vi "Analyze.vi"(8 "error in (no error)":errorcluster, 9 "Work Image":T1, 10 "Destination":refnum<class "Message Enqueuer.lvclass">, 11 "Analyze Data":T2) -> (0 "error out":errorcluster)   [LabVIEW 2014, in "Analyze Actor.lvlib" / "Analyze Actor.lvclass"]
uses:
  Analyze Actor.lvclass
  HIJ Vision Display/HIJ Vision Display/Analyze.ctl
  Abstract Messages/Publish Analyze Results Msg/Publish Analyze Results Msg.lvclass
  <vilib>/vision/Image Controls.llb/IMAQ Image.ctl
  Analyze Classes/Analyze BaseClass/Analyze BaseClass/Analyze BaseClass.lvclass
  Results and Overlays/Results Base/Analyze Results Base.lvclass
  <vilib>/ActorFramework/Message Enqueuer/Message Enqueuer.lvclass
  Abstract Messages/Publish Analyze Results Msg/Publish Analyze Results Msg.lvclass/Publish Analyze Results Msg.ctl
  <vilib>/ActorFramework/Message Enqueuer/Message Enqueuer.lvclass/Message Enqueuer.ctl
  <vilib>/ActorFramework/Message Enqueuer/Enqueue.vi
  <vilib>/ActorFramework/Message Priority Queue/Priority Enqueue.vi
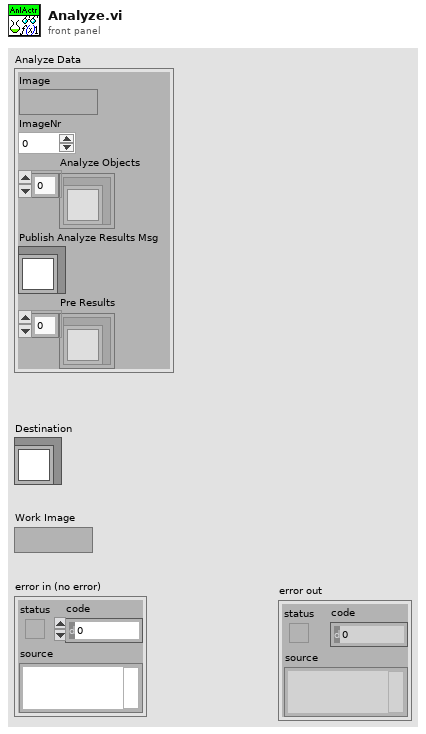
[diagram p1: front panel]
types:
  T1 = typedef "IMAQ Image.ctl" = refnum<image>
  T2 = typedef "Analyze Actor.lvlib/Analyze Actor.lvclass/Analyze.ctl" = cluster{"Image":T1, "ImageNr":i32, "Analyze Objects":refnum<class "Analyze BaseClass.lvclass">[], "Publish Analyze Results Msg":refnum<class "Publish Analyze Results Msg.lvclass">, "Pre Results":refnum<class "Analyze Results Base.lvclass">[]}
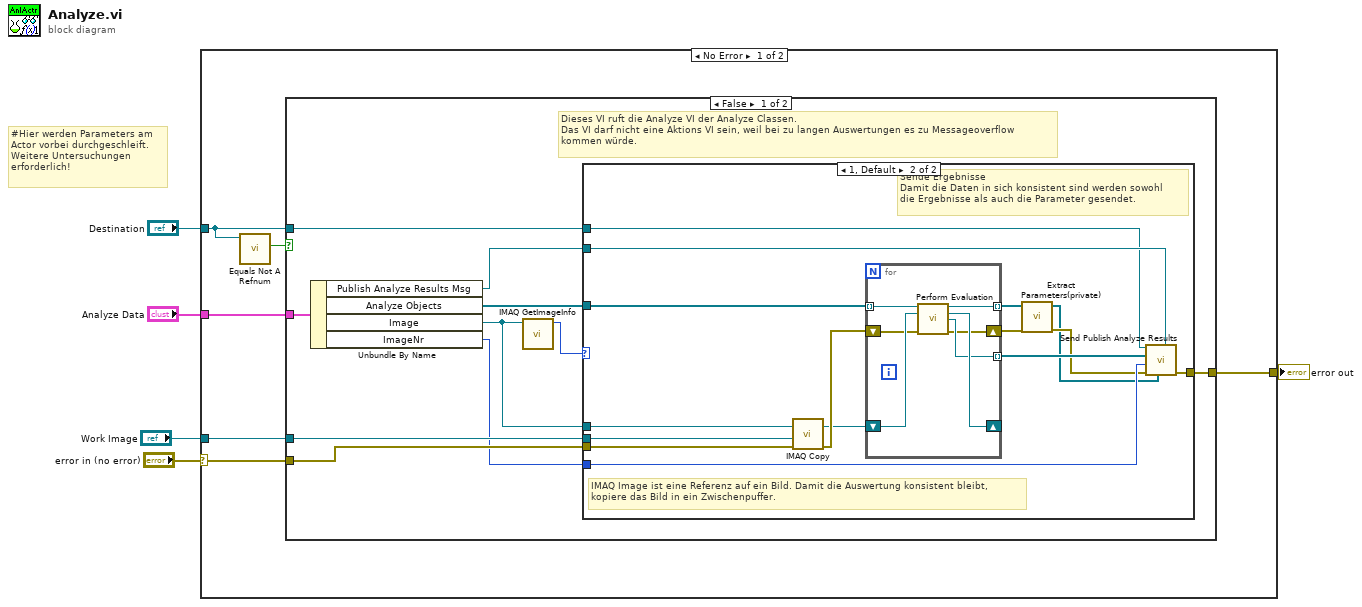
[diagram p0: block diagram]
diagram:
  # "#Hier werden Parameters am\nActor vorbei durchgeschleift.\nWeitere Untersuchungen \nerforderlich!"
  n1 = case shown="No Error" "error in (no error)" {
    selector: "error in (no error)" -> [w11 w46]
    tunnel: [w9 w46] -> w4
    tunnel: "Analyze Data" -> [w10 _]
    tunnel: "Destination" -> [w8 _]
    tunnel: "Work Image" -> [w6 _]
    frame No Error {
      n2 = call <vilib>:"Equals Not A Refnum.vi"("Message Enqueuer"=w8) -> ("Not a refnum?"=w7:bool)  [unwired: 10 in]
      n3 = case shown="False" w7 {
        tunnel: w11 -> [w15 w45]
        tunnel: w10 -> [w20 _]
        tunnel: [w18 w45] -> w9
        tunnel: w8 -> [w17 _]
        tunnel: w6 -> [w16 _]
        frame False {
          # "Dieses VI ruft die Analyze VI der Analyze Classen.\nDas VI darf nicht eine Aktions VI sein, weil bei zu langen Auswertungen es zu Messageoverflow\nkommen würde."
          n4 = Unbundle By Name(w20) -> ("Publish Analyze Results Msg"=w21:refnum<class "Publish Analyze Results Msg.lvclass">, "Analyze Objects"=w19:refnum<class "Analyze BaseClass.lvclass">[], "Image"=w13:T1, "ImageNr"=w14:i32)
          n5 = call "IMAQ GetImageInfo"("Image"=w13) -> ("X Resolution"=w12:i32)  [unwired: 3 in, 7 out]
          n6 = case shown="1, Default" w12 {
            tunnel: w21 -> [_ w37]
            tunnel: w19 -> [_ w36]
            tunnel: [w22 w35] -> w18
            tunnel: w17 -> [_ w34]
            tunnel: w16 -> [_ w33]
            tunnel: w15 -> [w22 w32]
            tunnel: w14 -> [_ w29]
            tunnel: w13 -> [_ w23]
            frame 0 {
            }
            frame 1, Default {
              # "Sende Ergebnisse\nDamit die Daten in sich konsistent sind werden sowohl\ndie Ergebnisse als auch die Parameter gesendet."
              # "IMAQ Image ist eine Referenz auf ein Bild. Damit die Auswertung konsistent bleibt,\nkopiere das Bild in ein Zwischenpuffer."
              n7 = call "IMAQ Copy"("error in (no error)"=w32, "Image Dst"=w33, "Image Src"=w23) -> ("error out"=w31:errorcluster, "Image Dst Out"=w30:T1)  [unwired: 3 in]
              n8 = for {
                tunnel: w36 -> [w43] mode=indexing
                shift-right: [w42] -> _
                shift-left: w30 -> [w44]
                shift-right: [w39] -> w26
                shift-left: w31 -> [w41]
                tunnel: [w40] -> w28 mode=indexing
                tunnel: [w38] -> w27 mode=indexing
                n9 = call "Perform Evaluation.vi"("Analyze BaseClass in"=w43, "Image in"=w44, "error in (no error)"=w41) -> ("Analyze BaseClass out"=w38:refnum<class "Analyze BaseClass.lvclass">, "Image out"=w42:T1, "Result"=w40:refnum<class "Analyze Results Base.lvclass">, "error out"=w39:errorcluster)  [unwired: 9 in]
              }
              n10 = call "Extract Parameters(private).vi"("error in"=w26, "Analyze objs"=w27) -> ("error out"=w25:errorcluster, "Parameters"=w24:refnum<class "Analyze Parameter Base.lvclass">[])  [unwired: 8 in]
              n11 = call "Send Publish Analyze Results.vi"("Message Type"=w37, "Parameters"=w24, "error in (no error)"=w25, "Image Nr."=w29, "Results In"=w28, "Message Enqueuer"=w34) -> ("error out"=w35:errorcluster)  [unwired: 4 in, 1 out]
            }
          }
        }
        frame True {
        }
      }
    }
    frame Error {
    }
  }
  "error out" <- w4
